vi "RefreshSystemConfigurationUI.vi"(8 "error in (no error)":errorcluster, 11 "SoftwareSetup in":refnum<class "SoftwareSetup.lvclass">) -> (0 "error out":errorcluster, 3 "SoftwareSetup out":refnum<class "SoftwareSetup.lvclass">)   [LabVIEW 2019, in "SoftwareSetup.lvlib" / "SoftwareSetup.lvclass"]
uses:
  SoftwareSetup.lvclass
  C:/Program Files (x86)/National Instruments/LabVIEW 2019/vi.lib/NI/Event Source Actor/Event Source/Event Source/Event Source.lvclass
  StationOptions.lvclass
  C:/Program Files (x86)/National Instruments/LabVIEW 2019/vi.lib/NI/Event Source Actor/Event Source/Event/Event.lvclass
  <vilib>/NI/Event Source Actor/Event Source/Event/Event.lvclass/Event.ctl
  SoftwareSetup.lvclass/SoftwareSetup.ctl
  SystemSetup/SystemSetup/SystemSetup.lvclass
  <vilib>/Utility/config.llb/NI_LVConfig.lvlib
  <vilib>/NI/Event Source Actor/Event Source/Event/Event.lvclass
  <vilib>/NI/Event Source Actor/Event Source/Event Source/Event Source.lvclass
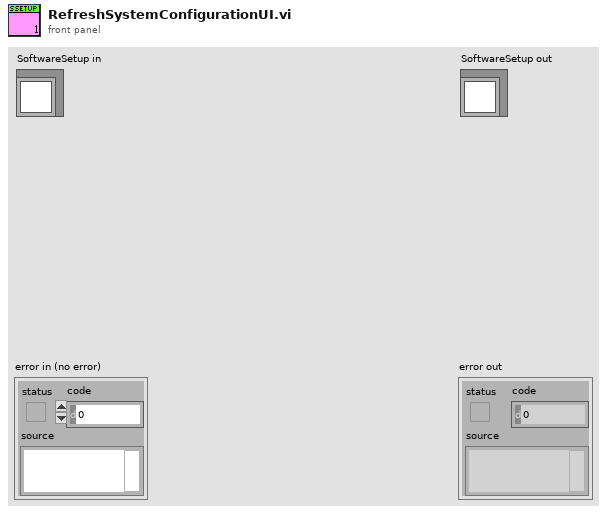
[diagram p1: front panel]
types:
  T1 = typedef "SoftwareSetup.lvlib/DataBase.ctl" = cluster{"Connection String Expression":string, "User ID":string, "Password":string}
  T2 = typedef "SoftwareSetup.lvlib/Local Report.ctl" = cluster{"Report Path":path, "Report  Format":enum16{"CSV", "XML", "PDF", "Excel", "TXT"}, "Disabled State":bool, "Customer name":string}
  T3 = typedef "SoftwareSetup.lvlib/Localization.ctl" = cluster{"Language":enum16{"English", "Chinese"}}
  T4 = typedef "SoftwareSetup.lvlib/Preferences.ctl" = cluster{"Station ID":string, "IP Address":string, "Password":string}
  T5 = typedef "SoftwareSetup.lvlib/User Manager.ctl" = cluster{"Current User Manager File":string, "Login on start":bool}
  T6 = typedef "SoftwareSetup.lvlib/Multiple UUT Settings.ctl" = cluster{"Number of Tests Sockets":u8, "Synchronization":enum16{"Don't Synchronize", "Serial", "Parallel", "One Thread Only"}}
  T7 = typedef "SoftwareSetup.lvlib/Sequence.ctl" = cluster{"Sequence Folder Path":path}
  T8 = cluster{"DataBase":T1, "Local Report":T2, "Localization":T3, "Preferences":T4, "User Manager":T5, "Multiple UUT Settings":T6, "Sequence":T7}
  T9 = typedef "NI_LVConfig.lvlib/Config Data RefNum.ctl" = refnum<k1>
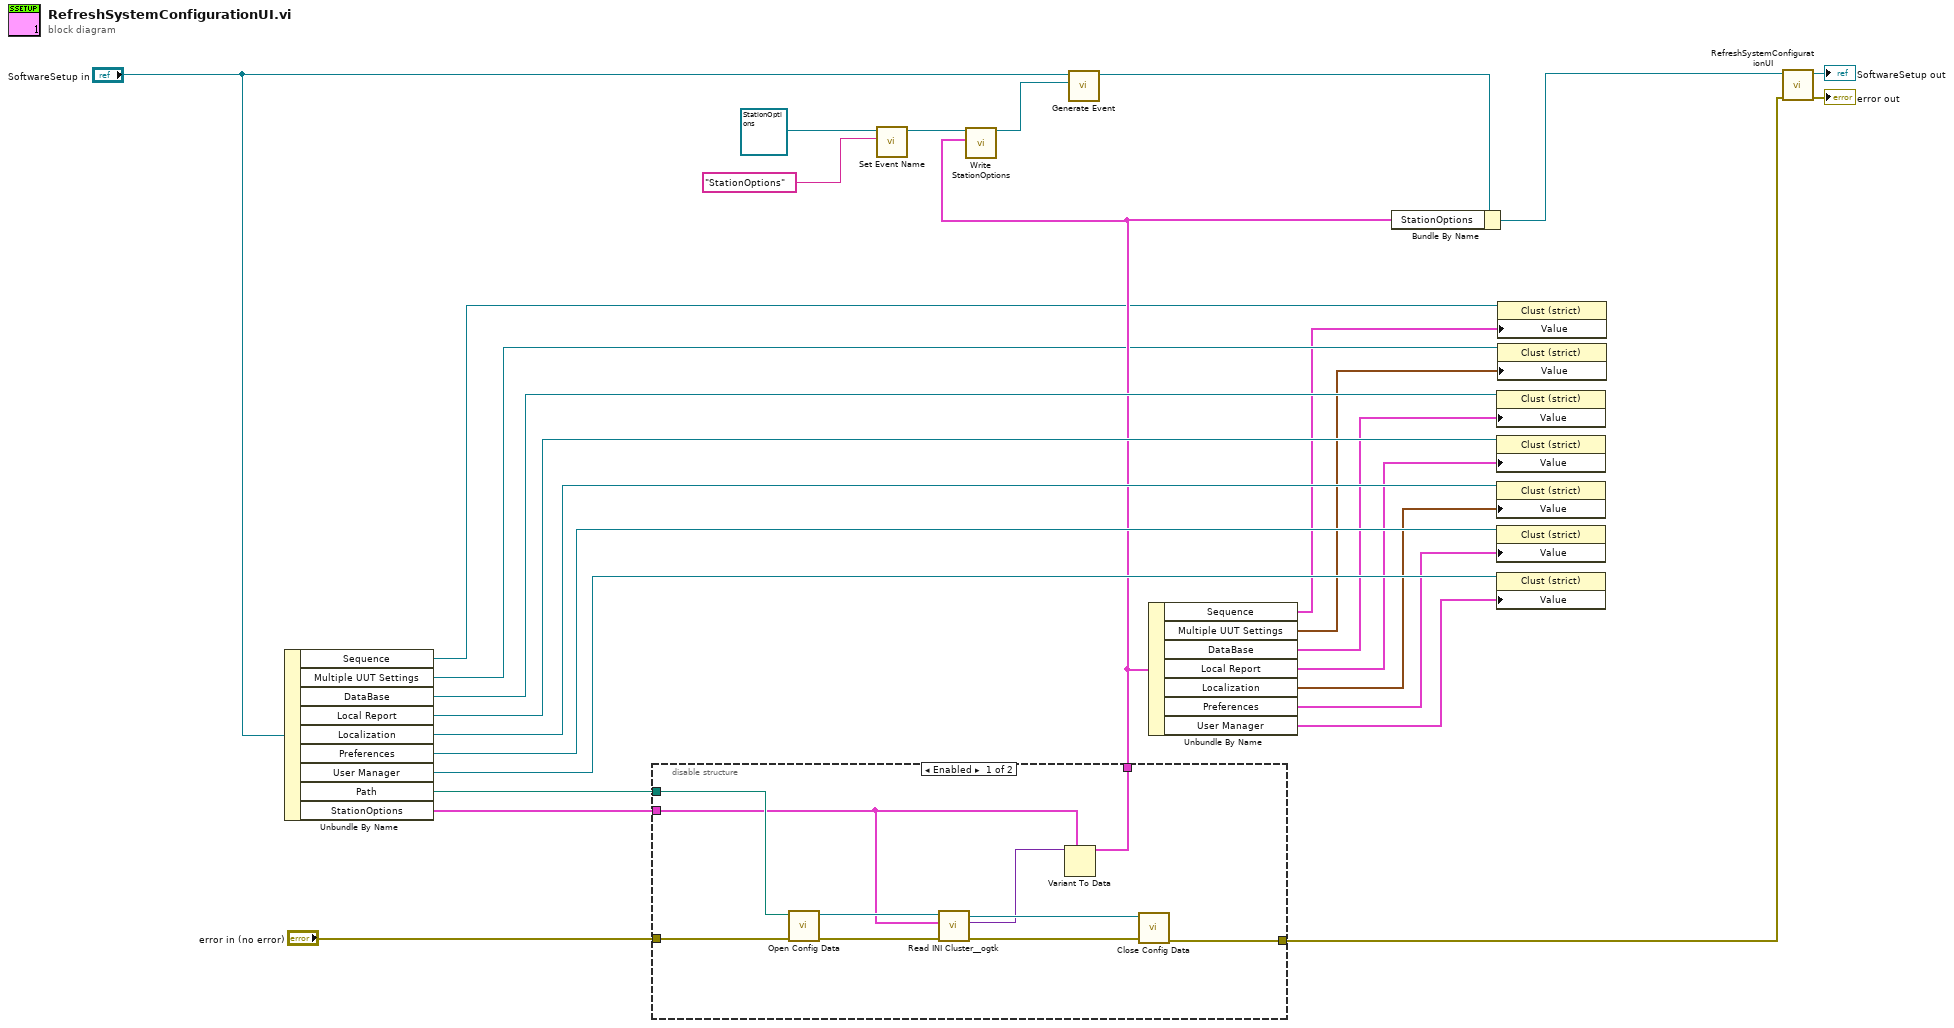
[diagram p0: block diagram]
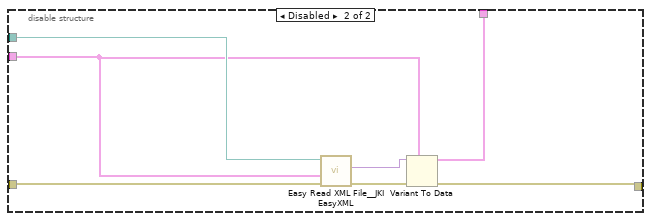
[diagram p2: hidden frame]
diagram:
  n1 = Unbundle By Name("SoftwareSetup in") -> ("Sequence"=w2:refnum<vi>, "Multiple UUT Settings"=w4:refnum<vi>, "DataBase"=w24:refnum<vi>, "Local Report"=w23:refnum<vi>, "Localization"=w22:refnum<vi>, "Preferences"=w21:refnum<vi>, "User Manager"=w20:refnum<vi>, "Path"=w26:path, "StationOptions"=w6:T8)
  n2 = disable-structure shown="Enabled" {
    disable-tunnel: w26 -> [w33 w44]
    disable-tunnel: "error in (no error)" -> [w32 w45]
    disable-tunnel: [w31 w39] -> w12
    disable-tunnel: [w30 w41] -> w7
    disable-tunnel: w6 -> [w29 w42]
    frame Enabled {
      n3 = call <vilib>:"Open Config Data.vi"("error in (no error)"=w32, "configuration file path"=w33) -> ("error out"=w37:errorcluster, "refnum"=w38:T9)  [unwired: 7 in, 1 out]
      n4 = call <userlib>:"Read INI Cluster__ogtk.vi"("error in (no error)"=w37, "INI Fomatted Cluster Type"=w29, "refnum"=w38) -> ("error out"=w35:errorcluster, "INI Fomatted Cluster"=w34:variant, "dup refnum"=w36:T9)  [unwired: 4 in, 2 out]
      n5 = Variant To Data(type=w29, Variant=w34) -> (data=w30:T8)  [unwired: 1 in, 1 out]
      n6 = call <vilib>:"Close Config Data.vi"("error in (no error)"=w35, "refnum"=w36) -> ("error out"=w31:errorcluster)  [unwired: 8 in, 1 out]
    }
    frame Disabled {
      n7 = call <vilib>:"Easy Read XML File__JKI EasyXML.vi"("error in (no error)"=w45, "LabVIEW Data (Type)"=w42, "XML File Path"=w44) -> ("error out"=w40:errorcluster, "LabVIEW Data"=w43:variant)  [unwired: 6 in, 1 out]
      n8 = Variant To Data(error in=w40, type=w42, Variant=w43) -> (data=w41:T8, error out=w39:errorcluster)
    }
  }
  n9 = call <vilib>:"Set Event Name.vi"("Name (Generic)"="StationOptions", "Event In"=refnum<class "StationOptions.lvclass"> refnum ("SoftwareSetup.lvlib:StationOptions.lvclass")) -> ("Event Out"=w8:refnum<class "StationOptions.lvclass">)  [unwired: 9 in]
  n10 = call-dynamic "Write StationOptions.vi"("StationOptions"=w7, "StationOptions in"=w8) -> ("StationOptions out"=w10:refnum<class "StationOptions.lvclass">)  [unwired: 8 in, 1 out]
  n11 = call <vilib>:"Generate Event.vi"("Event"=w10, "Event Source In"="SoftwareSetup in") -> ("Event Source Out"=w19:refnum<class "SoftwareSetup.lvclass">)  [unwired: 8 in, 1 out]
  n12 = Unbundle By Name(w7) -> ("Sequence"=w1:T7, "Multiple UUT Settings"=w3:T6, "DataBase"=w17:T1, "Local Report"=w16:T2, "Localization"=w15:T3, "Preferences"=w14:T4, "User Manager"=w13:T5)
  n13 = Bundle By Name(cluster=w19, "StationOptions"=w7) -> (w18:refnum<class "SoftwareSetup.lvclass">)
  n14 = property class="Clust (strict)"(reference=w24, "Value"=w17) -> ()  [unwired: 1 in, 2 out]
  n15 = property class="Clust (strict)"(reference=w23, "Value"=w16) -> ()  [unwired: 1 in, 2 out]
  n16 = property class="Clust (strict)"(reference=w22, "Value"=w15) -> ()  [unwired: 1 in, 2 out]
  n17 = property class="Clust (strict)"(reference=w21, "Value"=w14) -> ()  [unwired: 1 in, 2 out]
  n18 = property class="Clust (strict)"(reference=w20, "Value"=w13) -> ()  [unwired: 1 in, 2 out]
  n19 = property class="Clust (strict)"(reference=w2, "Value"=w1) -> ()  [unwired: 1 in, 2 out]
  n20 = property class="Clust (strict)"(reference=w4, "Value"=w3) -> ()  [unwired: 1 in, 2 out]
  n21 = call-parent "RefreshSystemConfigurationUI.vi"("error in (no error)"=w12, "SystemSetup in"=w18) -> ("error out"=→"error out":errorcluster, "SystemSetup out"=→"SoftwareSetup out":refnum<class "SoftwareSetup.lvclass">)  [unwired: 8 in]
